vi "OpenDOSession.vi"(8 "error in (no error)":errorcluster, 10 "gRPCid":T5, 11 "DIOSessions In":T1={"Array of DI Sessions"=[], "Array of DO Sessions"=[], "Stream ReadDI"={"gRPCid ReadDI"=0, "DISessionName"="", "Stream Status ReadDI"=FALSE, "Async Stop ReadDI Queue"=refnum, "DI Task"="", "ms to wait"=500}}) -> (0 "error out":errorcluster, 3 "DIOSessions Out":T1={"Array of DI Sessions"=[], "Array of DO Sessions"=[], "Stream ReadDI"={"gRPCid ReadDI"=0, "DISessionName"="", "Stream Status ReadDI"=FALSE, "Async Stop ReadDI Queue"=refnum, "DI Task"="", "ms to wait"=500}})   [LabVIEW 2019, in "ctet_dio_User Library.lvlib"]
uses:
  ctet_dio_User Library.lvlib
  Servers/ctet_dio/gRPC lvSupport/Server API/typeDefs/grpcId.ctl
  Types/DIOSessions.ctl
  Types/DISession.ctl
  Types/DOSession.ctl
  Types/StreamReadDI.ctl
  Servers/ctet_dio/ctet_dio Class/RPC Messages/measurementservice_DOOpenSessionResponse/measurementservice_DOOpenSessionResponse_Data.ctl
  Servers/ctet_dio/ctet_dio Class/RPC Messages/measurementservice_ErrorOut/measurementservice_ErrorOut_Data.ctl
  <vilib>/DAQmx/create/channels.llb/DAQmx Create Channel (DO-Digital Output).vi
  Servers/ctet_dio/ctet_dio Class/ctet_dio.lvclass
  Servers/ctet_dio/gRPC lvSupport/gprc-lvsupport.lvlib
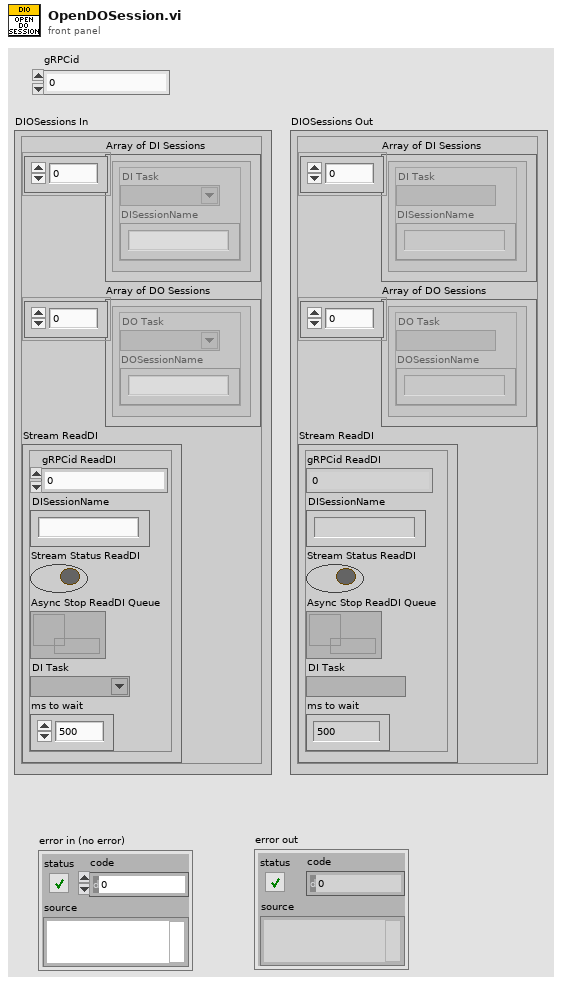
[diagram p1: front panel]
types:
  T1 = typedef "ctet_dio_User Library.lvlib/DIOSessions.ctl" = cluster{"Array of DI Sessions":T2[], "Array of DO Sessions":T3[], "Stream ReadDI":T4}
  T2 = typedef "ctet_dio_User Library.lvlib/DISession.ctl" = cluster{"DI Task":refnum<k21>, "DISessionName":string}
  T3 = typedef "ctet_dio_User Library.lvlib/DOSession.ctl" = cluster{"DO Task":refnum<k21>, "DOSessionName":string}
  T4 = typedef "ctet_dio_User Library.lvlib/StreamReadDI.ctl" = cluster{"gRPCid ReadDI":T5, "DISessionName":string, "Stream Status ReadDI":bool, "Async Stop ReadDI Queue":refnum<queue>, "DI Task":refnum<k21>, "ms to wait":u32}
  T5 = typedef "ctet_dio.lvlib/gprc-lvsupport.lvlib/grpcId.ctl" = u64
  T6 = typedef "ctet_dio.lvlib/ctet_dio.lvclass/measurementservice_ErrorOut_Data.ctl" = cluster{"errCode":i64, "errMessage":string}
  T7 = typedef "ctet_dio.lvlib/ctet_dio.lvclass/measurementservice_DOOpenSessionResponse_Data.ctl" = cluster{"DOSessionName":string, "error":T6}
  T8 = typedef "ctet_dio.lvlib/ctet_dio.lvclass/measurementservice_DOOpenSessionRequest_Data.ctl" = cluster{"DOSessionName":string, "DOlines":string}
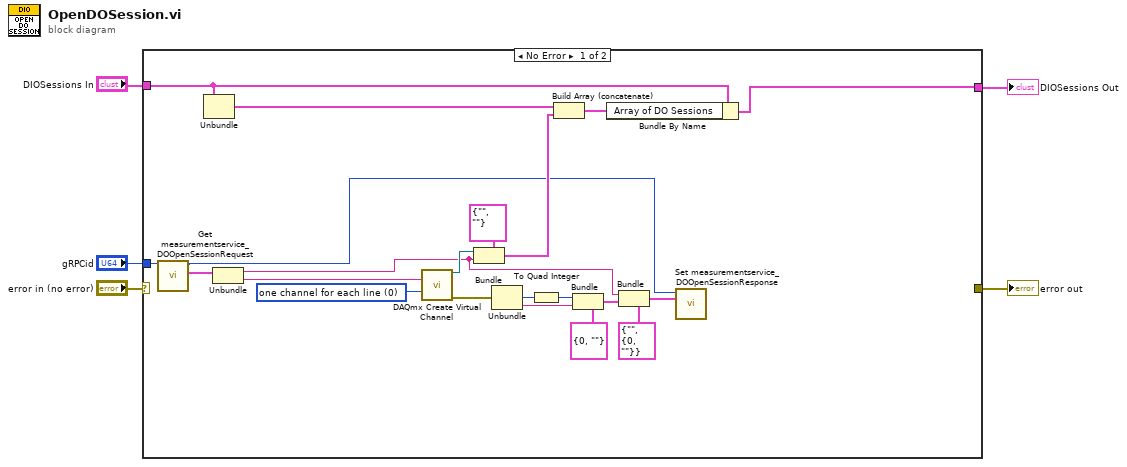
[diagram p0: block diagram]
diagram:
  n1 = case shown="No Error" "error in (no error)" {
    selector: "error in (no error)" -> [_ w28]
    tunnel: [_ w28] -> w5
    tunnel: "gRPCid" -> [w15 _]
    tunnel: "DIOSessions In" -> [w23 w27]
    tunnel: [w22 w27] -> w1
    frame No Error {
      w16 = 0 items=["one channel for each line", "one channel for all lines"] ("line grouping")
      n2 = call "Get measurementservice_DOOpenSessionRequest.vi"("gRPCid"=w15) -> ("Message Data"=w14:T8, "gRPCid out"=w9:T5)  [unwired: 8 in, 1 out]
      n3 = Unbundle(w23) -> ("Array of DO Sessions"=w11:T3[])  [unwired: 2 out]
      n4 = Unbundle(w14) -> ("DOSessionName"=w19:string, "DOlines"=w26:string)
      n5 = call-poly <vilib>:"DAQmx Create Virtual Channel.vi"("lines"=w26, "line grouping"=w16) -> ("task out"=w25:refnum<k21>, "error out"=w21:errorcluster)  [unwired: 12 in]
      n6 = Bundle(cluster=T3 {"DO Task"="", "DOSessionName"=""} ("DOSession"), "DO Task"=w25, "DOSessionName"=w19) -> (w12:T3)
      n7 = Unbundle(w21) -> ("code"=w18:i32, "source"=w20:string)  [unwired: 1 out]
      n8 = To Quad Integer(1:w18) -> (0:w17:i64)
      n9 = Build Array (concatenate)(w11, w12) -> (w24:T3[])
      n10 = Bundle(cluster=T6 {"errCode"=0, "errMessage"=""} ("error"), "errCode"=w17, "errMessage"=w20) -> (w6:T6)
      n11 = Bundle By Name(cluster=w23, "Array of DO Sessions"=w24) -> (w22:T1)
      n12 = Bundle(cluster=T7 {"DOSessionName"="", "error"={"errCode"=0, "errMessage"=""}} ("measurementservice_DOOpenSessionResponse_Data"), "DOSessionName"=w19, "error"=w6) -> (w8:T7)
      n13 = call "Set measurementservice_DOOpenSessionResponse.vi"("Message Data"=w8, "gRPCid"=w9) -> ()  [unwired: 9 in, 1 out]
    }
    frame Error {
    }
  }
  "error out" <- w5
  "DIOSessions Out" <- w1
